vi "Xilinx FFT.vi"(10 "sample timing":T3, 11 "channels in":T2) -> (1 "output valid":bool=TRUE, 2 "subcarrier channels":T1, 3 "OFDM symbol index":u16)   [LabVIEW 2020]
uses:
  <vilib>/rvi/DataTransferAndStorage/Container/Common/niFpgaContainerExecOnDevCompGetState.vi
  <vilib>/rvi/Emulation/niFpgaEmulationIsFPGAContextNoSignature.vi
  <vilib>/rvi/Emulation/niFpgaSctlEmulationGetInTimedLoop.vi
  <vilib>/rvi/errors/niFpgaSetErrorForExecOnDevCompSimple.vi
  <vilib>/rvi/eio/common/nirviEmuReportErrorAndStop.vi
  <vilib>/rvi/DataTransferAndStorage/Container/Common/niFpgaContainerGetUniqueNameForEmu.vi
  <vilib>/rvi/FIFO/Fifo_Resource/nirvififoEmulationSetSize.vi
  <vilib>/rvi/FIFO/Fifo_Resource/nirviFifoEmulationQueueMgr.vi
  <instcachedir>/0/nirviFifoEmulationQueueMgr_E5CAEC123FF24DC58D834DCA3CDAA9B5.lvgen/nirviFifoEmulationQueueMgr_E5CAEC123FF24DC58D834DCA3CDAA9B5_005.vi
  <vilib>/rvi/FIFO/Fifo_Resource/nirvififoEmulationDetermineInputValidOut.vi
  <vilib>/rvi/FIFO/Fifo_Resource/nirvififoEmulationCreateLock.vi
  <vilib>/rvi/Emulation/niFpgaProcessEmulError.vi
  <vilib>/rvi/FIFO/Fifo_Resource/nirvififoEmulationObtainLock.vi
  <vilib>/rvi/FIFO/Fifo_Resource/nirvififoEmulationReleaseLock.vi
  <vilib>/rvi/occurrence/nirviWaitOnOccurrenceBase.vi
  <vilib>/rvi/errors/nirviReportUnexpectedCaseInternalError.vi
  <vilib>/rvi/errors/nirviReportUnexpectedCaseInternalError (U32).vi
  <vilib>/Utility/error.llb/Clear Errors.vi
  <vilib>/rvi/interface/RandomDataEmulation/niFpgaRandomDataHandleErrors.vi
  <vilib>/rvi/DataTransferAndStorage/Container/XNode/niFpgaContainer.xnode
  <vilib>/rvi/FIFO/Fifo_Resource/niFpgaFifoEmulationRefIn.vi
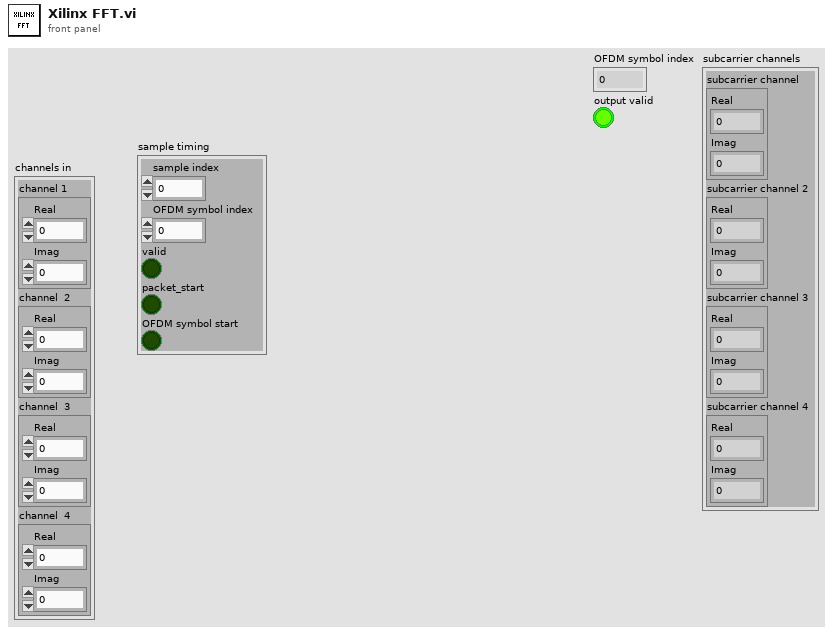
[diagram p1: front panel]
types:
  T1 = cluster{"subcarrier channel":cluster{"Real":fxp<+/-,25,4>, "Imag":fxp<+/-,25,4>}, "subcarrier channel 2":cluster{"Real":fxp<+/-,25,4>, "Imag":fxp<+/-,25,4>}, "subcarrier channel 3":cluster{"Real":fxp<+/-,25,4>, "Imag":fxp<+/-,25,4>}, "subcarrier channel 4":cluster{"Real":fxp<+/-,25,4>, "Imag":fxp<+/-,25,4>}}
  T2 = cluster{"channel 1 ":cluster{"Real":fxp<+/-,16,3>, "Imag":fxp<+/-,16,3>}, "channel  2":cluster{"Real":fxp<+/-,16,3>, "Imag":fxp<+/-,16,3>}, "channel  3":cluster{"Real":fxp<+/-,16,3>, "Imag":fxp<+/-,16,3>}, "channel  4":cluster{"Real":fxp<+/-,16,3>, "Imag":fxp<+/-,16,3>}}
  T3 = cluster{"sample index":u16, "OFDM symbol index":u16, "valid":bool, "packet_start":bool, "OFDM symbol start":bool}
  T4 = cluster{"Real":fxp<+/-,16,3>, "Imag":fxp<+/-,16,3>}
  T5 = cluster{"Real":fxp<+/-,25,4>, "Imag":fxp<+/-,25,4>}
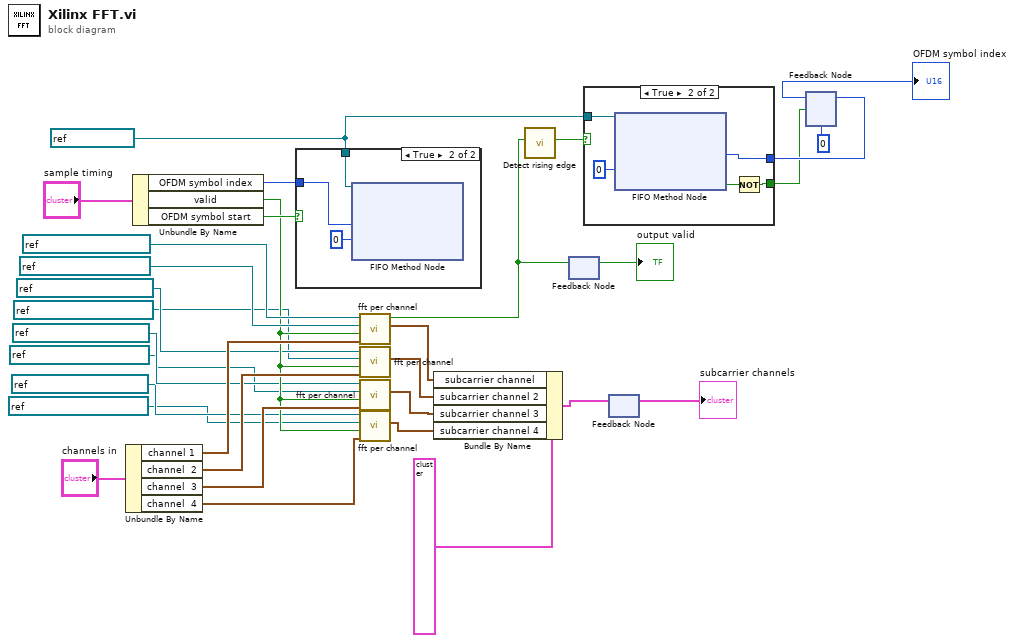
[diagram p0: block diagram]
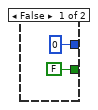
[diagram p2: hidden frame]
diagram:
  w19 = refnum<k21> "FFT FIFO U" ("FFT FIFO U In")
  n1 = Unbundle By Name("channels in") -> ("channel 1"=w17:T4, "channel  2"=w10:T4, "channel  3"=w9:T4, "channel  4"=w8:T4)
  n2 = Unbundle By Name("sample timing") -> ("OFDM symbol index"=w30:u16, "valid"=w7:bool, "OFDM symbol start"=w31:bool)
  n3 = case shown="True" w31 {
    tunnel: w30 -> [_ w35]
    tunnel: w19 -> [_ w33]
    frame False {
    }
    frame True {
      n4 = xnode ("FIFO Method Node")("Element"=w35, "Timeout"=0, "FIFO In"=w33) -> ()  [unwired: 2 out]
    }
  }
  n5 = call "fft per channel.vi"("sample in"=w17, "valid"=w7, "FIFO FFT CPX IMAG In"=refnum<k21> "FIFO FFT CPX IMAG", "FIFO FFT CPX REAL In"=refnum<k21> "FIFO FFT CPX REAL") -> ("sample out"=w14:T5, "m_axis_data_tvalid"=w23:bool)  [unwired: 6 in]
  n6 = call "fft per channel.vi"("sample in"=w10, "valid"=w7, "FIFO FFT CPX IMAG In"=refnum<k21> "FIFO FFT CPX 2 IMAG", "FIFO FFT CPX REAL In"=refnum<k21> "FIFO FFT CPX 2 REAL") -> ("sample out"=w13:T5)  [unwired: 6 in, 1 out]
  n7 = call "fft per channel.vi"("sample in"=w9, "valid"=w7, "FIFO FFT CPX IMAG In"=refnum<k21> "FIFO FFT CPX 3 IMAG", "FIFO FFT CPX REAL In"=refnum<k21> "FIFO FFT CPX 3 REAL") -> ("sample out"=w12:T5)  [unwired: 6 in, 1 out]
  n8 = call "fft per channel.vi"("sample in"=w8, "valid"=w7, "FIFO FFT CPX IMAG In"=refnum<k21> "FIFO FFT CPX 4 IMAG", "FIFO FFT CPX REAL In"=refnum<k21> "FIFO FFT CPX 4 REAL") -> ("sample out"=w11:T5)  [unwired: 6 in, 1 out]
  n9 = Bundle By Name(cluster=T1 {"subcarrier channel"={"Real"=0.0, "Imag"=0.0}, "subcarrier channel 2"={"Real"=0.0, "Imag"=0.0}, "subcarrier channel 3"={"Real"=0.0, "Imag"=0.0}, "subcarrier channel 4"={"Real"=0.0, "Imag"=0.0}}, "subcarrier channel"=w14, "subcarrier channel 2"=w13, "subcarrier channel 3"=w12, "subcarrier channel 4"=w11) -> (w15:T1)
  n10 = call "Detect rising edge.vi"("signal"=w23) -> ("edge detected"=w25:bool)  [unwired: 10 in]
  n11 = feedback-in #1(w23) -> ()
  n12 = feedback #1() -> (→"output valid":bool)  [unwired: 1 in]
  n13 = case shown="True" w25 {
    tunnel: [u16 0 ("Element") w41] -> w28
    tunnel: [FALSE w39] -> w26
    tunnel: w19 -> [_ w38]
    frame False {
    }
    frame True {
      n14 = xnode ("FIFO Method Node")("Timeout"=0, "FIFO In"=w38) -> ("Element"=w41:u16, "Timed Out?"=w40:bool)  [unwired: 1 out]
      n15 = Not(x=w40) -> (.not. x?=w39:bool)
    }
  }
  n16 = feedback #2() -> (→"subcarrier channels":T1)  [unwired: 1 in]
  n17 = feedback-in #2(w15) -> ()
  n18 = feedback-in #3(w28, w26) -> ()
  n19 = feedback #3(u16 0 ("Element")) -> (→"OFDM symbol index":u16)
